vi "testEvent.vi"() -> ()   [LabVIEW 2011]
panel:
  in  "Numeric":i32
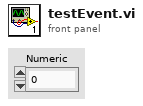
[diagram p1: front panel]
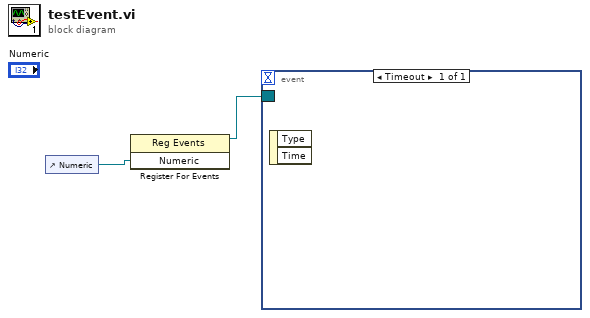
[diagram p0: block diagram]
diagram:
  n1 = control-ref of="Numeric"() -> (w2:refnum<vi>)
  n2 = register-events(w2) -> (reference out=w1:refnum<event-registration>)  [unwired: 2 in, 1 out]
  n3 = event shown="[0] Timeout" {
    selector: w1 -> [_]
    dyn-events: _ -> [_]
    timeout: _ -> [_]
    event Timeout {
      n4 = event-data() -> ()  [unwired: 1 in, 2 out]
    }
  }
